vi "Untitled5.vi"() -> ()   [LabVIEW 2020]
uses:
  HAL/Source/Communicator/Communicator.lvclass
  D:/git/HAL/Source/Interfaces/IInstrument/IInstrument.lvclass
  D:/git/HAL/Source/Interfaces/IClose/IClose.lvclass
  D:/git/HAL/Source/Interfaces/IInitialize/IInitialize.lvclass
  D:/git/HAL/Source/Communicator/Communicator.lvclass
  D:/git/HAL/Source/Interfaces/ICommunicate/ICommunicate.lvclass
  D:/git/HAL/Source/Interfaces/IConfigurable/IConfigurable.lvclass
  D:/git/HAL/Source/Interfaces/IRunnable/IRunnable.lvclass
  D:/git/HAL/Source/Interfaces/IUnmanaged/IUnmanaged.lvclass
  CANopen Master/CANopen Master.lvclass
  <vilib>/ProgressBar/Progress Bar Dialog.lvclass
  EDS-File-Viewer/source/Electronic Datasheet/Electronic Datasheet.lvclass
  source/Object Dictionary/Object Dictionary.lvclass
  source/Object Entry/Object Entry.lvclass
  source/Sub Object/Sub Object.lvclass
panel:
  out "Success":bool[](array[boolean])
  out "Objects List":string[](array[string])
  out "Values":variant[](array[variant])
  in  "Actual Values Button":bool
  out "Uploaded":variant
  out "MSG Log":string
  in  "Discover Button":bool
  out "Success? DL":bool
  in  "Value":u16
  in  "Multiplexer DL":cluster{"Index":u16, "Sub-Index":u8} {"Index" format="%.0x"}
  in  "Download Button":bool
  in  "Node-ID DL":u8
  out "Available Nodes":map{u8, u8}(c390)
  out "Success? UL":bool
  out "Data UL":u8[](array[numeric]) format="%.0x"
  in  "Node-ID UPL":u8
  in  "Multiplexer":cluster{"Index":u16, "Sub-Index":u8} {"Index" format="%.0x"}
  in  "Upload Button":bool
  out "Emergency?":bool[](array[boolean])
  out "Nodes":u8[](array[numeric])
  in  "stop":bool
  out "Timed Outs?":bool[](array[boolean])
  out "Node-IDs":u8[](array[numeric])
  out "error out":errorcluster
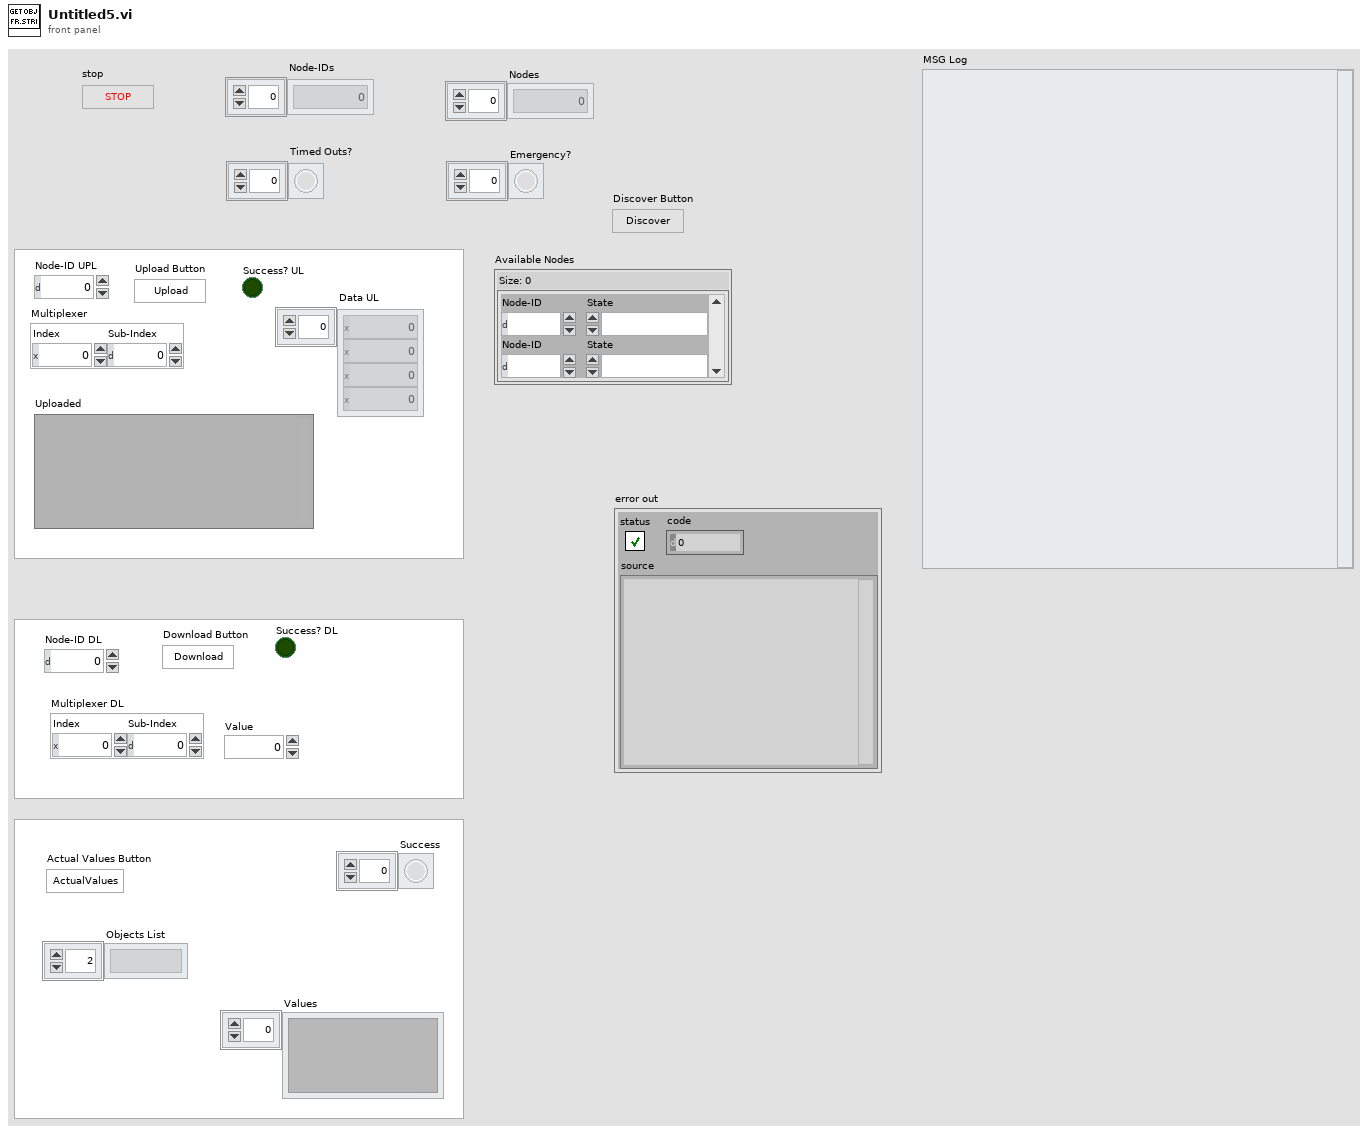
[diagram p1: front panel]
types:
  T1 = cluster{"CAN Task":cluster{"Stop":refnum<user-event>, "Msg Received":refnum<user-event>, "Error":refnum<user-event>}, "NMT":cluster{"Node Discovered":refnum<user-event>}, "Heartbeat Producer":cluster{"Stop":refnum<user-event>, "Error":refnum<user-event>}}
  T2 = typedef "CANopen.lvlib/SDO Result.ctl" = cluster{"Success":bool, "SDO abort code":cluster{"Null":bool, "Value":T3}, "Data":cluster{"Null":bool, "Data":u8[]}}
  T3 = typedef "CANopen Master.lvlib/SDO Transfer.lvclass/SDO abort code.ctl" = u32
  T4 = typedef "CANopen.lvlib/Data Type.ctl" = u16
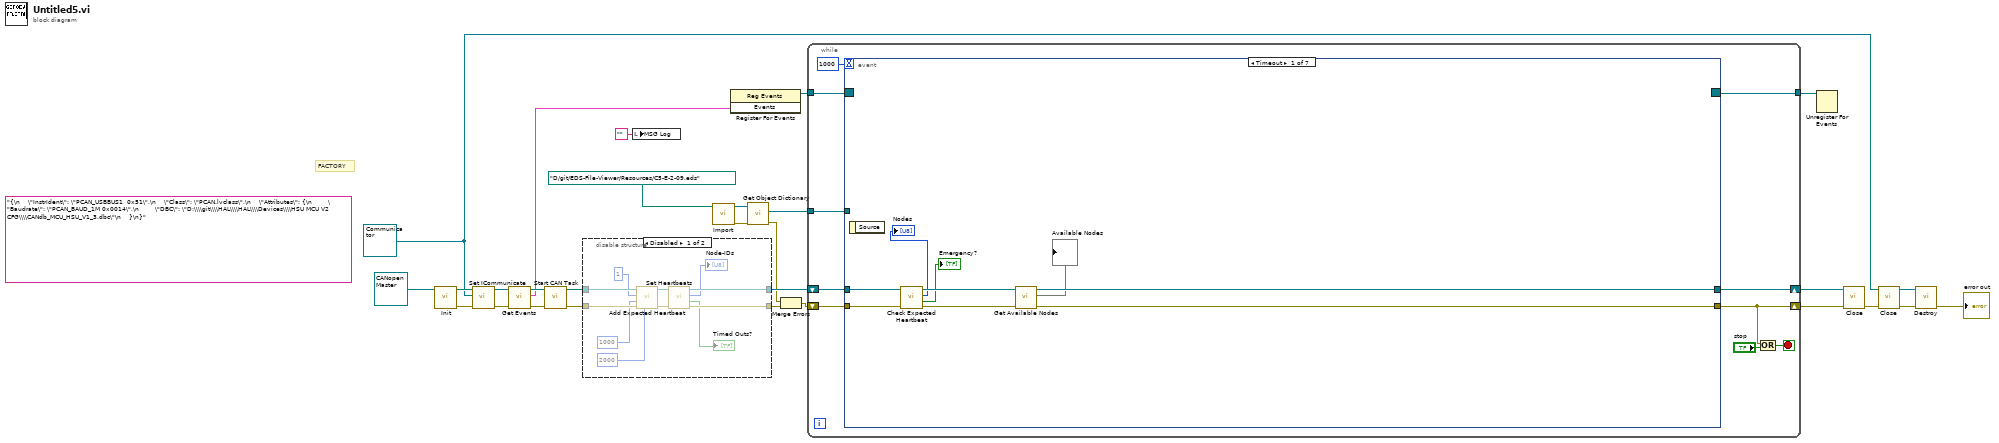
[diagram p0: block diagram]
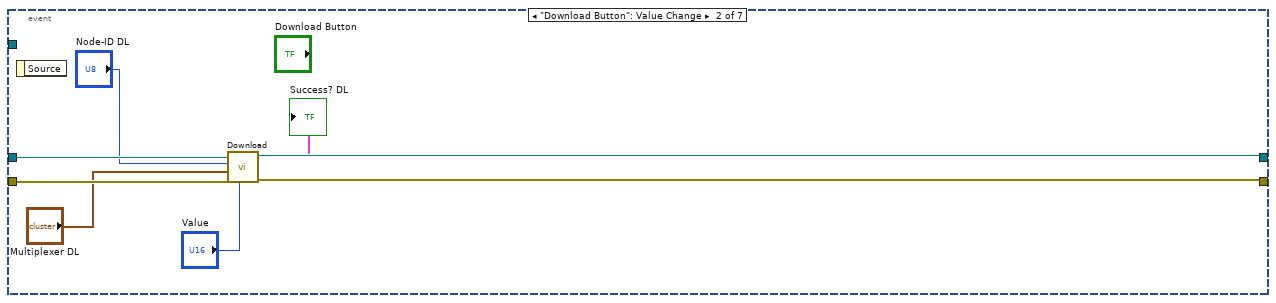
[diagram p3: hidden frame]
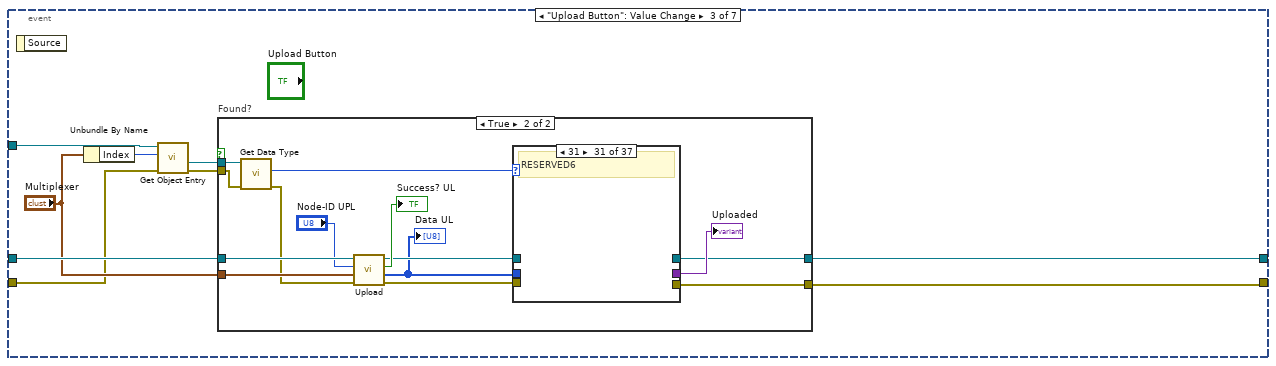
[diagram p4: hidden frame]
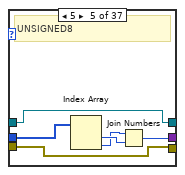
[diagram p10: hidden frame]
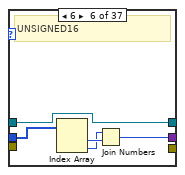
[diagram p11: hidden frame]
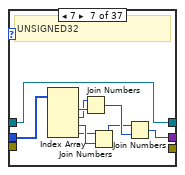
[diagram p12: hidden frame]
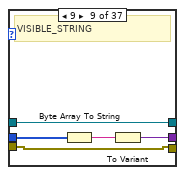
[diagram p14: hidden frame]
diagram:
  w10 = refnum<class "Communicator.lvclass"> refnum ("Communicator")
  (unwired) "{\n    \"InstrIdent\": \"PCAN_USBBUS1  0x51\",\n    \"Class\": \"PCAN.lvclass\",\n    \"Attributes\": {\n        \"Baudrate\": \"PCAN_BAUD_1M 0x0014\",\n        \"DBC\": \"D:\\\\git\\\\HAL\\\\HAL\\\\Devices\\\\HSU MCU V2 CFG\\\\CANdb_MCU_HSU_V1_3.dbc\"\n    }\n}" ("<JSON>CFG")
  # "FACTORY"
  n1 = call "Init.vi"("CANopen Master in"=refnum<class "CANopen Master.lvclass"> refnum ("CANopen Master.lvlib:CANopen Master")) -> ("error out"=w23:errorcluster, "CANopen Master out"=w24:refnum<class "CANopen Master.lvclass">)  [unwired: 9 in]
  n2 = call "Set ICommunicate.vi"("ICommunicate"=w10, "CANopen Master in"=w24) -> ("CANopen Master out"=w12:refnum<class "CANopen Master.lvclass">)  [unwired: 8 in, 1 out]
  n3 = call "Get Events.vi"("CANopen Master in"=w12) -> ("Events"=w5:T1, "CANopen Master out"=w11:refnum<class "CANopen Master.lvclass">)  [unwired: 8 in, 1 out]
  n4 = call "Start CAN Task.vi"("error in"=w23, "CANopen Master in"=w11) -> ("error out"=w16:errorcluster, "CANopen Master out"=w15:refnum<class "CANopen Master.lvclass">)  [unwired: 8 in]
  n5 = disable-structure shown="Disabled" {
    disable-tunnel: w16 -> [w37 w38]
    disable-tunnel: w15 -> [w36 w39]
    disable-tunnel: [w35 w39] -> w22
    disable-tunnel: [w34 w38] -> w21
    frame Disabled {
      n6 = call "Add Expected Heartbeat.vi"("Timeout"=u16 2000, "error in"=w37, "Period"=u16 1000, "Node-ID"=u8 1, "CANopen Master in"=w36) -> ("error out"=w30:errorcluster, "CANopen Master out"=w29:refnum<class "CANopen Master.lvclass">)  [unwired: 5 in]
      n7 = call "Set Heartbeats.vi"("error in"=w30, "CANopen Master in"=w29) -> ("error out"=w34:errorcluster, "Timed Outs?"=→"Timed Outs?":bool[], "Node-IDs"=→"Node-IDs":u8[], "CANopen Master out"=w35:refnum<class "CANopen Master.lvclass">)  [unwired: 6 in]
    }
    frame Enabled {
    }
  }
  n8 = local write "MSG Log"("") -> ()
  n9 = call "Import.vi"("EDS File Path"=path "D:/git/EDS-File-Viewer/Resources/C5-E-2-09.eds") -> ("error out"=w4:errorcluster, "Electronic Datasheet"=w3:refnum<class "Electronic Datasheet.lvclass">)  [unwired: 9 in]
  n10 = register-events(w5) -> (reference out=w14:refnum<event-registration>)  [unwired: 2 in, 1 out]
  n11 = call "Get Object Dictionary.vi"("error in"=w4, "Electronic Datasheet in"=w3) -> ("error out"=w2:errorcluster, "Obj Dict"=w1:refnum<class "Object Dictionary.lvclass">)  [unwired: 7 in, 1 out]
  n12 = Merge Errors(w2, w21) -> (w17:errorcluster)
  n13 = while {
    shift-right: [w46] -> w19
    shift-left: w22 -> [w48]
    shift-right: [w45] -> w20
    shift-left: w17 -> [w47]
    tunnel: w14 -> [w42]
    tunnel: [w41] -> w13
    tunnel: w1 -> [w40]
    stop <- w44 stop-if-true
    n14 = event shown="[0] Timeout" {
      selector: w42 -> [_ _ _ _ _ _ _]
      dyn-events: [_ _ _ _ _ _ _] -> w41
      timeout: 1000 -> [_ _ _ _ _ _ _]
      tunnel: w48 -> [w56 w64 w74 w130 w226 w233 w241]
      tunnel: w47 -> [w57 w65 w68 w131 w227 w234 w242]
      tunnel: [w55 w63 w72 w122 w227 w234 w240] -> w45
      tunnel: [w51 w62 w71 w119 w226 w233 w239] -> w46
      tunnel: w40 -> [_ _ w66 w118 _ _ _]
      event Timeout {
        n15 = event-data() -> ()  [unwired: 1 in, 1 out]
        n16 = call "Check Expected Heartbeat.vi"("error in"=w57, "CANopen Master in"=w56) -> ("error out"=w55:errorcluster, "Emergency?"=→"Emergency?":bool[], "Nodes"=→"Nodes":u8[], "CANopen Master out"=w54:refnum<class "CANopen Master.lvclass">)  [unwired: 6 in]
        n17 = call "Get Available Nodes.vi"("CANopen Master in"=w54) -> ("Nodes"=→"Available Nodes":map{u8, u8}, "CANopen Master out"=w51:refnum<class "CANopen Master.lvclass">)  [unwired: 8 in, 1 out]
      }
      event "Download Button": Value Change {
        n18 = event-data() -> ()  [unwired: 1 in, 1 out]
        n19 = call "Download.vi"("Value"="Value", "error in"=w65, "Multiplexer"="Multiplexer DL", "Node-ID"="Node-ID DL", "CANopen Master in"=w64) -> ("error out"=w63:errorcluster, "SDO Result"=→"Success? DL":T2, "CANopen Master out"=w62:refnum<class "CANopen Master.lvclass">)  [unwired: 4 in]
      }
      event "Upload Button": Value Change {
        n20 = event-data() -> ()  [unwired: 1 in, 1 out]
        n21 = Unbundle By Name("Multiplexer") -> ("Index"=w70:u16)
        n22 = call "Get Object Entry.vi"("error in"=w68, "OD Index"=w70, "Obj Dict in"=w66) -> ("error out"=w67:errorcluster, "Obj Entry"=w69:refnum<class "Object Entry.lvclass">)  [unwired: 6 in, 1 out]
        n23 = case "Found?" shown="True" {
          selector: _ -> [_ _]
          tunnel: w74 -> [w76 w90]
          tunnel: "Multiplexer" -> [_ w89]
          tunnel: [w75 w82] -> w72
          tunnel: [w76 w81] -> w71
          tunnel: w69 -> [_ w80]
          tunnel: w67 -> [w75 w79]
          frame False {
          }
          frame True {
            n24 = call "Get Data Type.vi"("error in"=w79, "Object Entry in"=w80) -> ("error out"=w77:errorcluster, "Data Type"=w87:T4)  [unwired: 7 in, 1 out]
            n25 = call "Upload.vi"("error in"=w77, "Multiplexer"=w89, "Node-ID"="Node-ID UPL", "CANopen Master in"=w90) -> ("error out"=w85:errorcluster, "Value"=w84:u8[], "Success?"=→"Success? UL":bool, "CANopen Master out"=w86:refnum<class "CANopen Master.lvclass">)  [unwired: 4 in]
            "Data UL" <- w84
            n26 = case shown="31" w87 {
              tunnel: w86 -> [_ _ _ _ w95 w97 w102 _ w112 _ _ _ _ _ _ _ _ _ _ _ _ _ _ _ _ _ _ _ _ _ _ _ _ _ _ _ w117]
              tunnel: w85 -> [_ _ _ _ w91 _ _ _ w113 _ _ _ _ _ _ _ _ _ _ _ _ _ _ _ _ _ _ _ _ _ _ _ _ _ _ _ w116]
              tunnel: w84 -> [_ _ _ _ w96 w101 w110 _ w115 _ _ _ _ _ _ _ _ _ _ _ _ _ _ _ _ _ _ _ _ _ _ _ _ _ _ _ _]
              tunnel: [_ _ _ _ w92 w98 w103 _ w111 _ _ _ _ _ _ _ _ _ _ _ _ _ _ _ _ _ _ _ _ _ _ _ _ _ _ _ _] -> w83
              tunnel: [_ _ _ _ w91 _ _ _ w113 _ _ _ _ _ _ _ _ _ _ _ _ _ _ _ _ _ _ _ _ _ _ _ _ _ _ _ w116] -> w82
              tunnel: [_ _ _ _ w95 w97 w102 _ w112 _ _ _ _ _ _ _ _ _ _ _ _ _ _ _ _ _ _ _ _ _ _ _ _ _ _ _ w117] -> w81
              frame 1 {
                # "BOOLEAN"
              }
              frame 2 {
                # "INTEGER8"
              }
              frame 3 {
                # "INTEGER16"
              }
              frame 4 {
                # "INTEGER32"
              }
              frame 5 {
                # "UNSIGNED8"
                n27 = Index Array(array=w96) -> (element #1=w94:u8, element #2=w93:u8)  [unwired: 2 in]
                n28 = Join Numbers(hi=w93, lo=w94) -> ((hi.lo)=w92:u16)
              }
              frame 6 {
                # "UNSIGNED16"
                n29 = Index Array(array=w101) -> (element #1=w100:u8, element #2=w99:u8)  [unwired: 2 in]
                n30 = Join Numbers(hi=w99, lo=w100) -> ((hi.lo)=w98:u16)
              }
              frame 7 {
                # "UNSIGNED32"
                n31 = Index Array(array=w110) -> (element #1=w109:u8, element #2=w108:u8, element #3=w107:u8, element #4=w106:u8)  [unwired: 4 in]
                n32 = Join Numbers(hi=w108, lo=w109) -> ((hi.lo)=w105:u16)
                n33 = Join Numbers(hi=w106, lo=w107) -> ((hi.lo)=w104:u16)
                n34 = Join Numbers(hi=w104, lo=w105) -> ((hi.lo)=w103:u32)
              }
              frame 8 {
                # "REAL32"
              }
              frame 9 {
                # "VISIBLE_STRING"
                n35 = Byte Array To String(unsigned byte array=w115) -> (string=w114:string)
                n36 = To Variant(anything=w114) -> (Variant=w111:variant)
              }
              frame 10 {
                # "OCTET_STRING"
              }
              frame 11 {
                # "UNICODE_STRING"
              }
              frame 12 {
                # "TIME_OF_DAY"
              }
              frame 13 {
                # "TIME_DIFFERENCE"
              }
              frame 14 {
                # "RESERVED1"
              }
              frame 15 {
                # "DOMAIN"
              }
              frame 16 {
                # "INTEGER24"
              }
              frame 17 {
                # "REAL64"
              }
              frame 18 {
                # "INTEGER40"
              }
              frame 19 {
                # "INTEGER48"
              }
              frame 20 {
                # "INTEGER56"
              }
              frame 21 {
                # "INTEGER64"
              }
              frame 22 {
                # "UNSIGNED24"
              }
              frame 23 {
                # "RESERVED2"
              }
              frame 24 {
                # "UNSIGNED40"
              }
              frame 25 {
                # "UNSIGNED48"
              }
              frame 26 {
                # "UNSIGNED56"
              }
              frame 27 {
                # "UNSIGNED64"
              }
              frame 28 {
                # "RESERVED3"
              }
              frame 29 {
                # "RESERVED4"
              }
              frame 30 {
                # "RESERVED5"
              }
              frame 31 {
                # "RESERVED6"
              }
              frame 32 {
                # "PDO_COMMUNICATION_PARAMETER"
              }
              frame 33 {
                # "PDO_MAPPING"
              }
              frame 34 {
                # "SDO_PARAMETER"
              }
              frame 35 {
                # "IDENTITY"
              }
              frame 36 {
                # "RESERVED7"
              }
              frame Default {
                # "INVALID"
              }
            }
            "Uploaded" <- w83
          }
        }
      }
      event "Actual Values Button": Value Change {
        n37 = event-data() -> ()  [unwired: 1 in, 1 out]
        n38 = call "Get Communication Profile Objects.vi"("error in"=w131, "Obj Dict in"=w118) -> ("error out"=w124:errorcluster, "Communcation Profile"=w121:refnum<class "Object Entry.lvclass">[])  [unwired: 7 in, 1 out]
        n39 = local read "Node-ID UPL"() -> (w123:u8)
        n40 = Array Size(array=w121) -> (size(s)=w127:i32)
        n41 = call <vilib>:"Launch Progress Bar.vi"("Main Title (\"Working...\")"="Uploading Actual Values" ("Main Title (\"Working...\")"), "Total Count"=w127) -> ("Progress Bar Dialog"=w129:refnum<class "Progress Bar Dialog.lvclass">)  [unwired: 8 in, 1 out]
        n42 = for {
          tunnel: w121 -> [w139] mode=indexing
          shift-right: [w145] -> w128
          shift-left: w129 -> [w146]
          tunnel: [w147] -> w125 mode=concatenating
          shift-right: [w144] -> w119
          shift-left: w130 -> [w148]
          tunnel: w123 -> [w143]
          shift-right: [w142] -> w122
          shift-left: w124 -> [w138]
          tunnel: [w140] -> w120 mode=concatenating
          n43 = property class="Obj Entry"(reference=w139, error in=w138) -> (reference out=w134:refnum<class "Object Entry.lvclass">, error out=w137:errorcluster, "Index"=w132:u16, "Sub Objects"=w135:refnum<class "Sub Object.lvclass">[])
          n44 = Format Into String(format string="0x%x", w132) -> (resulting string=w133:string)  [unwired: 2 in, 1 out]
          n45 = call <vilib>:"Increment Progress Bar.vi"("Step Name (\"\")"=w133, "Progress Bar Dialog in"=w146) -> ("Progress Bar Dialog out"=w145:refnum<class "Progress Bar Dialog.lvclass">)  [unwired: 7 in, 2 out]
          n46 = Array Size(array=w135) -> (size(s)=w141:i32)
          n47 = case "Index has Sub-Entries?" shown="0" w141 {
            tunnel: w148 -> [w164 w192]
            tunnel: [w160 w187] -> w147
            tunnel: w137 -> [w158 w189]
            tunnel: [w159 w191] -> w144
            tunnel: w143 -> [w161 w190]
            tunnel: [w152 w188] -> w142
            tunnel: w135 -> [_ w186]
            tunnel: [w156 w185] -> w140
            tunnel: w134 -> [w155 _]
            tunnel: w132 -> [w150 w184]
            frame 0 {
              n48 = Bundle("Index"=w150, u8 0) -> (w151:cluster{"Index":u16, u8})  [unwired: 1 in]
              n49 = call "Upload.vi"("error in"=w158, "Multiplexer"=w151, "Node-ID"=w161, "CANopen Master in"=w164) -> ("error out"=w153:errorcluster, "Value"=w163:u8[], "Success?"=w157:bool, "CANopen Master out"=w159:refnum<class "CANopen Master.lvclass">)  [unwired: 4 in]
              n50 = call "Get Data Type.vi"("error in"=w153, "Object Entry in"=w155) -> ("error out"=w152:errorcluster, "Data Type"=w154:T4)  [unwired: 7 in, 1 out]
              n51 = case shown="7" w154 {
                tunnel: w163 -> [_ _ _ _ w168 w172 w180 _ w183 _ _ _ _ _ _ _ _ _ _ _ _ _ _ _ _ _ _ _ _ _ _ _ _ _ _ _ _]
                tunnel: [_ _ _ _ w165 w169 w173 _ w181 _ _ _ _ _ _ _ _ _ _ _ _ _ _ _ _ _ _ _ _ _ _ _ _ _ _ _ _] -> w162
                frame 1 {
                  # "BOOLEAN"
                }
                frame 2 {
                  # "INTEGER8"
                }
                frame 3 {
                  # "INTEGER16"
                }
                frame 4 {
                  # "INTEGER32"
                }
                frame 5 {
                  # "UNSIGNED8"
                  n52 = Index Array(array=w168) -> (element #1=w167:u8, element #2=w166:u8)  [unwired: 2 in]
                  n53 = Join Numbers(hi=w166, lo=w167) -> ((hi.lo)=w165:u16)
                }
                frame 6 {
                  # "UNSIGNED16"
                  n54 = Index Array(array=w172) -> (element #1=w171:u8, element #2=w170:u8)  [unwired: 2 in]
                  n55 = Join Numbers(hi=w170, lo=w171) -> ((hi.lo)=w169:u16)
                }
                frame 7 {
                  # "UNSIGNED32"
                  n56 = Index Array(array=w180) -> (element #1=w179:u8, element #2=w178:u8, element #3=w177:u8, element #4=w176:u8)  [unwired: 4 in]
                  n57 = Join Numbers(hi=w178, lo=w179) -> ((hi.lo)=w175:u16)
                  n58 = Join Numbers(hi=w176, lo=w177) -> ((hi.lo)=w174:u16)
                  n59 = Join Numbers(hi=w174, lo=w175) -> ((hi.lo)=w173:u32)
                }
                frame 8 {
                  # "REAL32"
                }
                frame 9 {
                  # "VISIBLE_STRING"
                  n60 = Byte Array To String(unsigned byte array=w183) -> (string=w182:string)
                  n61 = To Variant(anything=w182) -> (Variant=w181:variant)
                }
                frame 10 {
                  # "OCTET_STRING"
                }
                frame 11 {
                  # "UNICODE_STRING"
                }
                frame 12 {
                  # "TIME_OF_DAY"
                }
                frame 13 {
                  # "TIME_DIFFERENCE"
                }
                frame 14 {
                  # "RESERVED1"
                }
                frame 15 {
                  # "DOMAIN"
                }
                frame 16 {
                  # "INTEGER24"
                }
                frame 17 {
                  # "REAL64"
                }
                frame 18 {
                  # "INTEGER40"
                }
                frame 19 {
                  # "INTEGER48"
                }
                frame 20 {
                  # "INTEGER56"
                }
                frame 21 {
                  # "INTEGER64"
                }
                frame 22 {
                  # "UNSIGNED24"
                }
                frame 23 {
                  # "RESERVED2"
                }
                frame 24 {
                  # "UNSIGNED40"
                }
                frame 25 {
                  # "UNSIGNED48"
                }
                frame 26 {
                  # "UNSIGNED56"
                }
                frame 27 {
                  # "UNSIGNED64"
                }
                frame 28 {
                  # "RESERVED3"
                }
                frame 29 {
                  # "RESERVED4"
                }
                frame 30 {
                  # "RESERVED5"
                }
                frame 31 {
                  # "RESERVED6"
                }
                frame 32 {
                  # "PDO_COMMUNICATION_PARAMETER"
                }
                frame 33 {
                  # "PDO_MAPPING"
                }
                frame 34 {
                  # "SDO_PARAMETER"
                }
                frame 35 {
                  # "IDENTITY"
                }
                frame 36 {
                  # "RESERVED7"
                }
                frame Default {
                  # "INVALID"
                }
              }
              n62 = Build Array(w157) -> (w156:bool[])
              n63 = Build Array(w162) -> (w160:variant[])
            }
            frame Default {
              n64 = for {
                shift-right: [w205] -> w191
                shift-left: w192 -> [w206]
                tunnel: w190 -> [w204]
                shift-right: [w199] -> w188
                shift-left: w189 -> [w203]
                tunnel: w186 -> [w195] mode=indexing
                tunnel: [w201] -> w187 mode=indexing
                tunnel: [w200] -> w185 mode=indexing
                tunnel: w184 -> [w197]
                n65 = property class="Sub Obj"(reference=w195, error in=w203) -> (error out=w196:errorcluster, "Sub Index"=w194:u8, "Data Type"=w193:T4)  [unwired: 1 out]
                n66 = Bundle("Index"=w197, "Sub Index"=w194) -> (w198:cluster{"Index":u16, "Sub Index":u8})  [unwired: 1 in]
                n67 = call "Upload.vi"("error in"=w196, "Multiplexer"=w198, "Node-ID"=w204, "CANopen Master in"=w206) -> ("error out"=w199:errorcluster, "Value"=w202:u8[], "Success?"=w200:bool, "CANopen Master out"=w205:refnum<class "CANopen Master.lvclass">)  [unwired: 4 in]
                n68 = case shown="7" w193 {
                  tunnel: w202 -> [_ _ _ _ w210 w214 w222 _ w225 _ _ _ _ _ _ _ _ _ _ _ _ _ _ _ _ _ _ _ _ _ _ _ _ _ _ _ _]
                  tunnel: [_ _ _ _ w207 w211 w215 _ w223 _ _ _ _ _ _ _ _ _ _ _ _ _ _ _ _ _ _ _ _ _ _ _ _ _ _ _ _] -> w201
                  frame 1 {
                    # "BOOLEAN"
                  }
                  frame 2 {
                    # "INTEGER8"
                  }
                  frame 3 {
                    # "INTEGER16"
                  }
                  frame 4 {
                    # "INTEGER32"
                  }
                  frame 5 {
                    # "UNSIGNED8"
                    n69 = Index Array(array=w210) -> (element #1=w209:u8, element #2=w208:u8)  [unwired: 2 in]
                    n70 = Join Numbers(hi=w208, lo=w209) -> ((hi.lo)=w207:u16)
                  }
                  frame 6 {
                    # "UNSIGNED16"
                    n71 = Index Array(array=w214) -> (element #1=w213:u8, element #2=w212:u8)  [unwired: 2 in]
                    n72 = Join Numbers(hi=w212, lo=w213) -> ((hi.lo)=w211:u16)
                  }
                  frame 7 {
                    # "UNSIGNED32"
                    n73 = Index Array(array=w222) -> (element #1=w221:u8, element #2=w220:u8, element #3=w219:u8, element #4=w218:u8)  [unwired: 4 in]
                    n74 = Join Numbers(hi=w220, lo=w221) -> ((hi.lo)=w217:u16)
                    n75 = Join Numbers(hi=w218, lo=w219) -> ((hi.lo)=w216:u16)
                    n76 = Join Numbers(hi=w216, lo=w217) -> ((hi.lo)=w215:u32)
                  }
                  frame 8 {
                    # "REAL32"
                  }
                  frame 9 {
                    # "VISIBLE_STRING"
                    n77 = Byte Array To String(unsigned byte array=w225) -> (string=w224:string)
                    n78 = To Variant(anything=w224) -> (Variant=w223:variant)
                  }
                  frame 10 {
                    # "OCTET_STRING"
                  }
                  frame 11 {
                    # "UNICODE_STRING"
                  }
                  frame 12 {
                    # "TIME_OF_DAY"
                  }
                  frame 13 {
                    # "TIME_DIFFERENCE"
                  }
                  frame 14 {
                    # "RESERVED1"
                  }
                  frame 15 {
                    # "DOMAIN"
                  }
                  frame 16 {
                    # "INTEGER24"
                  }
                  frame 17 {
                    # "REAL64"
                  }
                  frame 18 {
                    # "INTEGER40"
                  }
                  frame 19 {
                    # "INTEGER48"
                  }
                  frame 20 {
                    # "INTEGER56"
                  }
                  frame 21 {
                    # "INTEGER64"
                  }
                  frame 22 {
                    # "UNSIGNED24"
                  }
                  frame 23 {
                    # "RESERVED2"
                  }
                  frame 24 {
                    # "UNSIGNED40"
                  }
                  frame 25 {
                    # "UNSIGNED48"
                  }
                  frame 26 {
                    # "UNSIGNED56"
                  }
                  frame 27 {
                    # "UNSIGNED64"
                  }
                  frame 28 {
                    # "RESERVED3"
                  }
                  frame 29 {
                    # "RESERVED4"
                  }
                  frame 30 {
                    # "RESERVED5"
                  }
                  frame 31 {
                    # "RESERVED6"
                  }
                  frame 32 {
                    # "PDO_COMMUNICATION_PARAMETER"
                  }
                  frame 33 {
                    # "PDO_MAPPING"
                  }
                  frame 34 {
                    # "SDO_PARAMETER"
                  }
                  frame 35 {
                    # "IDENTITY"
                  }
                  frame 36 {
                    # "RESERVED7"
                  }
                  frame Default {
                    # "INVALID"
                  }
                }
              }
            }
          }
        }
        "Values" <- w125
        "Success" <- w120
        n79 = call <vilib>:"Close Progress Bar.vi"("Progress Bar Dialog"=w128) -> ()  [unwired: 10 in, 1 out]
      }
      event User Event {
        n80 = event-data() -> ("status"=w231:bool, "code"=w230:i32, "source"=w229:string)  [unwired: 1 in]
        n81 = Bundle By Name(cluster=errorcluster {"status"=FALSE, "code"=0, "source"=""} ("error constant"), "status"=w231, "code"=w230, "source"=w229) -> (w228:errorcluster)
        n82 = call <vilib>:"Simple Error Handler.vi"("error in (no error)"=w228) -> ()  [unwired: 4 in, 5 out]
      }
      event User Event {
        n83 = event-data() -> ("Message"=w235:string)  [unwired: 1 in]
        n84 = local read "MSG Log"() -> (w237:string)
        n85 = Concatenate Strings(w235, "\r", w237) -> (→"MSG Log":string)
      }
      event "Discover Button": Value Change {
        n86 = event-data() -> ()  [unwired: 1 in, 1 out]
        n87 = call "Discover Nodes.vi"("error in"=w242, "CANopen Master in"=w241) -> ("error out"=w240:errorcluster, "CANopen Master out"=w239:refnum<class "CANopen Master.lvclass">)  [unwired: 8 in]
      }
    }
    n88 = Or(x=w45, y="stop") -> (x .or. y?=w44:bool)
  }
  n89 = Unregister For Events(event registration refnum=w13) -> ()  [unwired: 1 in, 1 out]
  n90 = call "Close.vi"("error in"=w20, "CANopen Master in"=w19) -> ("error out"=w25:errorcluster)  [unwired: 8 in, 1 out]
  n91 = call-dynamic "Close.vi"("Error In"=w25, "Communicator in"=w10) -> ("Error Out"=w8:errorcluster, "Communicator out"=w9:refnum<class "Communicator.lvclass">)  [unwired: 8 in]
  n92 = call-dynamic "Destroy.vi"("Error In"=w8, "Communicator in"=w9) -> ("Error Out"=→"error out":errorcluster)  [unwired: 8 in, 1 out]
